vi "Stop Core.vi"(10 "final error code":i32, 11 "SkynetCompiler in":refnum<class "LVAutomationListener.lvclass">) -> (3 "SkynetCompiler out":refnum<class "LVAutomationListener.lvclass">)   [LabVIEW 2013, in "LVAutomationListener.lvlib" / "LVAutomationListener.lvclass"]
uses:
  LVAutomationListener.lvclass
  LVAutomationListener.lvclass/LVAutomationListener.ctl
  <vilib>/ActorFramework/Stop Msg/Stop Msg.lvclass/Stop Msg.ctl
  <vilib>/ActorFramework/Message Enqueuer/Message Enqueuer.lvclass/Message Enqueuer.ctl
  <vilib>/ActorFramework/Actor/Actor.lvclass
  <vilib>/ActorFramework/Stop Msg/Send Emergency Stop.vi
  <vilib>/ActorFramework/Stop Msg/Send Normal Stop.vi
  <vilib>/ActorFramework/Message Enqueuer/Enqueue Critical.vi
  <vilib>/ActorFramework/Message Enqueuer/Enqueue.vi
  <vilib>/ActorFramework/Message Priority Queue/Priority Enqueue.vi
  <vilib>/ActorFramework/Stop Msg/Stop Msg.lvclass
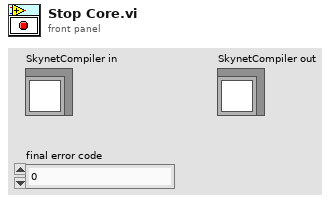
[diagram p1: front panel]
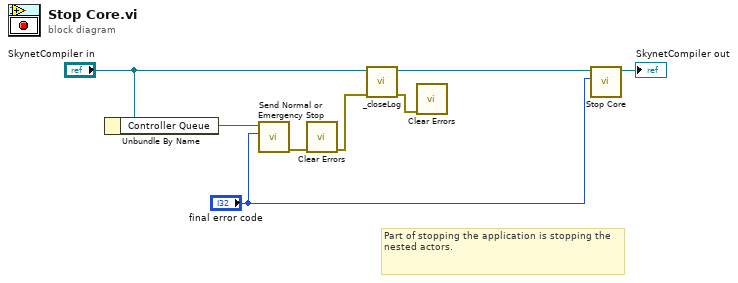
[diagram p0: block diagram]
diagram:
  # "Part of stopping the application is stopping the nested actors."
  n1 = Unbundle By Name("SkynetCompiler in") -> ("Controller Queue"=w5:refnum<class "Message Enqueuer.lvclass">)
  n2 = call <vilib>:"Send Normal or Emergency Stop.vi"("final error code"="final error code", "Message Enqueuer"=w5) -> ("error out"=w3:errorcluster)  [unwired: 9 in]
  n3 = call <vilib>:"Clear Errors.vi"("error in (no error)"=w3) -> ("error out"=w1:errorcluster)  [unwired: 6 in]
  n4 = call "_closeLog.vi"("error in (no error)"=w1, "SkynetCompiler in"="SkynetCompiler in") -> ("error out"=w7:errorcluster, "SkynetCompiler out"=w6:refnum<class "LVAutomationListener.lvclass">)  [unwired: 8 in]
  n5 = call <vilib>:"Clear Errors.vi"("error in (no error)"=w7) -> ()  [unwired: 6 in, 1 out]
  n6 = call-parent "Stop Core.vi"("final error code"="final error code", "Actor in"=w6) -> ("Actor out"=→"SkynetCompiler out":refnum<class "LVAutomationListener.lvclass">)  [unwired: 9 in]
